vi "close.vi"(8 "error in (no error)":errorcluster, 11 "VISA resource name":refnum<visa-resource-name>) -> (0 "error out":errorcluster)   [LabVIEW 2012]
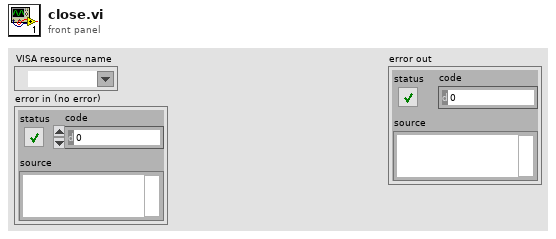
[diagram p1: front panel]
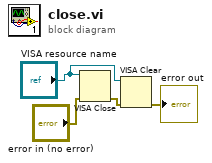
[diagram p0: block diagram]
diagram:
  n1 = VISA Close(VISA resource name="VISA resource name", error in (no error)="error in (no error)") -> (error out=w2:errorcluster)
  n2 = VISA Clear(VISA resource name="VISA resource name", error in (no error)=w2) -> (error out=→"error out":errorcluster)  [unwired: 1 out]
